vi "removePubSub.vi"(2 "Direction":enum16{"Publisher", "Subscriber"}(ring)=enum."Subscriber", 3 "PubSub":T1, 4 "ROS_Master in":refnum<class "ROS_Master.lvclass">) -> (0 "error out":errorcluster, 1 "ROS_Master out":refnum<class "ROS_Master.lvclass">)   [LabVIEW 2012, in "ROS_Master.lvclass"]
doc: "Try to unregister specified subscriber from the master. Throw error if unable to."
uses:
  ROS_Master.lvclass
  ROS_Master.lvclass/ROS_Master.ctl
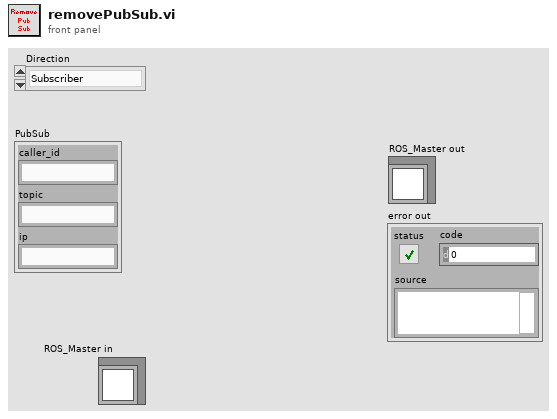
[diagram p1: front panel]
types:
  T1 = cluster{"caller_id":string, "topic":string, "ip":string}
  T2 = cluster{"Name":string, "PubSubs":cluster{"Caller ID":string, "IP":string, "Msg Type":string, "Direction":enum16{"Publisher", "Subscriber"}, "Topic":string}[]}[]
  T3 = cluster{"Name":string, "PubSubs":cluster{"Caller ID":string, "IP":string, "Msg Type":string, "Direction":enum16{"Publisher", "Subscriber"}, "Topic":string}[]}
  T4 = cluster{"Caller ID":string, "IP":string, "Msg Type":string, "Direction":enum16{"Publisher", "Subscriber"}, "Topic":string}[]
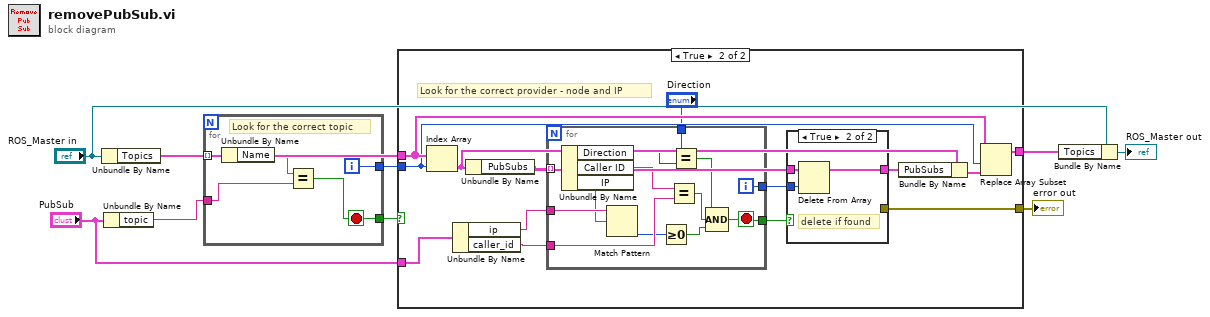
[diagram p0: block diagram]
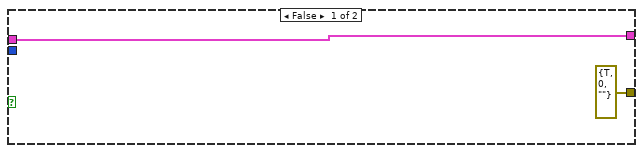
[diagram p2: hidden frame]
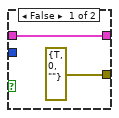
[diagram p3: hidden frame]
diagram:
  n1 = Unbundle By Name("ROS_Master in") -> ("Topics"=w8:T2)
  n2 = Unbundle By Name("PubSub") -> ("topic"=w9:string)
  n3 = for {
    tunnel: w8 -> [w14] mode=indexing
    tunnel: w9 -> [w12]
    tunnel: [w11] -> w7
    tunnel: [w10] -> w5
    i -> [w11]
    stop <- w10 stop-if-true
    # "Look for the correct topic"
    n4 = Unbundle By Name(w14) -> ("Name"=w13:string)
    n5 = Equal?(x=w13, y=w12) -> (x = y?=w10:bool)
  }
  n6 = case shown="True" w5 {
    tunnel: w8 -> [w16 w22]
    tunnel: w7 -> [_ w19]
    tunnel: "PubSub" -> [_ w30]
    tunnel: [w16 w20] -> w3
    tunnel: [errorcluster {"status"=TRUE, "code"=0, "source"=""} ("error constant") w18] -> w1
    frame False {
    }
    frame True {
      # "Look for the correct provider - node and IP"
      n7 = Index Array(array=w22, index=w19) -> (element=w24:T3)
      n8 = Unbundle By Name(w30) -> ("ip"=w28:string, "caller_id"=w29:string)
      n9 = Unbundle By Name(w24) -> ("PubSubs"=w27:T4)
      n10 = for {
        tunnel: w27 -> [w48] mode=indexing
        tunnel: w29 -> [w46]
        tunnel: w28 -> [w45]
        tunnel: [w38] -> w26
        tunnel: [w42] -> w25
        tunnel: "Direction" -> [w36]
        i -> [w42]
        stop <- w38 stop-if-true
        n11 = Unbundle By Name(w48) -> ("Direction"=w37:enum16{"Publisher", "Subscriber"}, "Caller ID"=w47:string, "IP"=w44:string)
        n12 = Match Pattern(string=w45, regular expression=w44) -> (offset past match=w43:i32)  [unwired: 1 in, 3 out]
        n13 = Greater Or Equal To 0?(x=w43) -> (x >= 0?=w41:bool)
        n14 = Equal?(x=w47, y=w46) -> (x = y?=w40:bool)
        n15 = Equal?(x=w36, y=w37) -> (x = y?=w39:bool)
        n16 = Compound Arithmetic op=AND(w39, w40, w41) -> (w38:bool)
      }
      n17 = case shown="True" w26 {
        tunnel: w27 -> [w32 w35]
        tunnel: w25 -> [_ w34]
        tunnel: [w32 w33] -> w23
        tunnel: [errorcluster {"status"=TRUE, "code"=0, "source"=""} ("error constant") _] -> w18
        frame False {
        }
        frame True {
          # "delete if found"
          n18 = Delete From Array(array=w35, index=w34) -> (array with subset deleted=w33:T4)  [unwired: 1 in, 1 out]
        }
      }
      n19 = Bundle By Name(cluster=w24, "PubSubs"=w23) -> (w21:T3)
      n20 = Replace Array Subset(array=w22, new element=w21, index=w19) -> (w20:T2)
    }
  }
  "error out" <- w1
  n21 = Bundle By Name(cluster="ROS_Master in", "Topics"=w3) -> (→"ROS_Master out":refnum<class "ROS_Master.lvclass">)
